vi "Plug Ins Main Cluster.vi"() -> (0 "Cluster":T1)   [LabVIEW 2011]
doc: "This is the cluster for both the main example and the challenge solution.\n\nAAL 9/09"
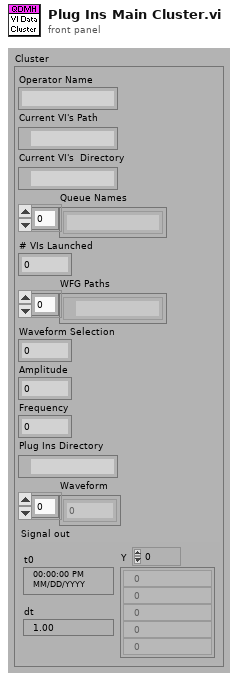
[diagram p1: front panel]
types:
  T1 = cluster{"Operator Name":string, "Current VI's Path":path, "Current VI's  Directory":path, "Queue Names":string[], "# VIs Launched":i32, "WFG Paths":path[], "Waveform Selection":i32, "Amplitude":dbl, "Frequency":dbl, "Plug Ins Directory":path, "Waveform":dbl[], "Signal out":waveform(dbl)}
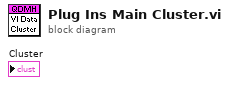
[diagram p0: block diagram]
diagram:
